vi "Write Time Stamp.vi"(8 "error in (no error)":errorcluster, 10 "Time Stamp":timestamp, 11 "time in":refnum<class "Timestamp.lvclass">) -> (0 "error out":errorcluster, 3 "time out":refnum<class "Timestamp.lvclass">)   [LabVIEW 2020, in "Example Source.lvlib" / "Timestamp.lvclass"]
uses:
  Timestamp.lvclass
  Timestamp.lvclass/Timestamp.ctl
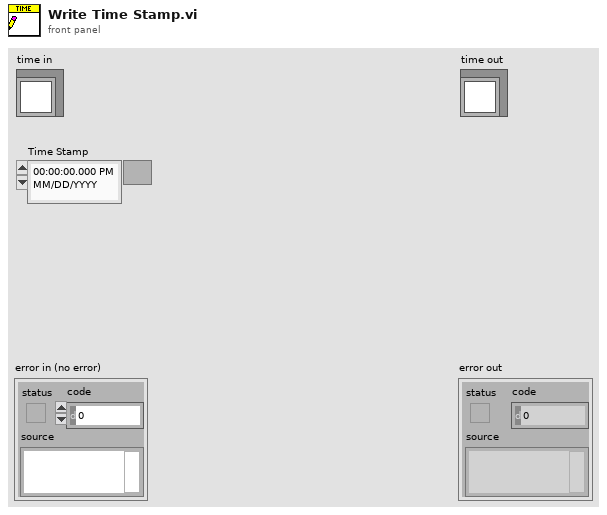
[diagram p1: front panel]
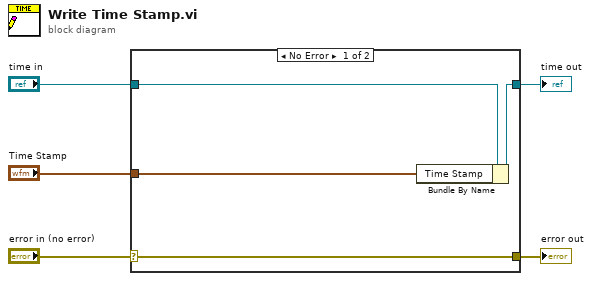
[diagram p0: block diagram]
diagram:
  n1 = case shown="No Error" "error in (no error)" {
    selector: "error in (no error)" -> [w9 w10]
    tunnel: [w9 w10] -> w4
    tunnel: [w7 w11] -> w2
    tunnel: "time in" -> [w8 w11]
    tunnel: "Time Stamp" -> [w6 _]
    frame No Error {
      n2 = Bundle By Name(cluster=w8, "Time Stamp"=w6) -> (w7:refnum<class "Timestamp.lvclass">)
    }
    frame Error {
    }
  }
  "error out" <- w4
  "time out" <- w2
